vi "Get Data from FIFO.vi"(7 "FIFO In":refnum<k21>="FIFOtoFFTLoop", 8 "Get New Data":bool, 11 "FFT State Info":T1) -> (0 "Data Valid":bool, 1 "Data":u32, 3 "FFT State Info Out":T1)   [LabVIEW 2011]
uses:
  <vilib>/rvi/DataTransferAndStorage/Container/Common/niFpgaContainerExecOnDevCompGetState.vi
  <vilib>/rvi/FIFO/Fifo_Resource/nirvififoEmulationSetSize.vi
  <vilib>/rvi/DataTransferAndStorage/Container/Common/niFpgaContainerGetUniqueNameForEmu.vi
  <vilib>/rvi/interface/RandomDataEmulation/nirviRandomDataFPGAFIFO.vi
  <vilib>/rvi/interface/RandomDataEmulation/niFpgaRandomDataHandleErrors.vi
  <vilib>/rvi/eio/common/nirviEmuReportErrorAndStop.vi
  <vilib>/rvi/FXPMathLib/basic elements/FxpDiscreteDelay/XNode/nifxpmath_DiscreteDelay.xnode
  <vilib>/rvi/DataTransferAndStorage/Container/XNode/niFpgaContainer.xnode
  <vilib>/rvi/FIFO/Fifo_Resource/niFpgaFifoEmulationRefIn.vi
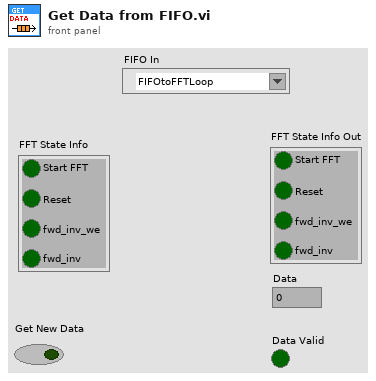
[diagram p1: front panel]
types:
  T1 = cluster{"Reset":bool, "Start FFT":bool, "fwd_inv_we":bool, "fwd_inv":bool}
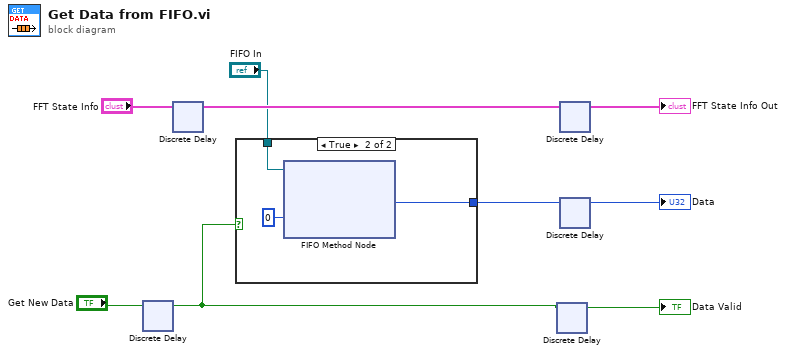
[diagram p0: block diagram]
diagram:
  n1 = xnode "Discrete Delay"("D"="Get New Data") -> ("Q"=w3:bool)
  n2 = xnode "Discrete Delay"("D"="FFT State Info") -> ("Q"=w7:T1)
  n3 = case shown="True" w3 {
    tunnel: [_ w10] -> w6
    tunnel: "FIFO In" -> [_ w12]
    frame False {
    }
    frame True {
      n4 = xnode ("FIFO Method Node")("Timeout"=0, "FIFO In"=w12) -> ("Element"=w10:u32)  [unwired: 2 out]
    }
  }
  n5 = xnode "Discrete Delay"("D"=w3) -> ("Q"=→"Data Valid":bool)
  n6 = xnode "Discrete Delay"("D"=w7) -> ("Q"=→"FFT State Info Out":T1)
  n7 = xnode "Discrete Delay"("D"=w6) -> ("Q"=→"Data":u32)
